vi "svx_DAQ_UpdateMenu.vi"(0 "MenuRef":refnum<k9>, 5 "Display State In":T1={"Channel Info Array"=[], "Timing Mode"=enum."Time", "Timing Control 1"=25600.0, "Timing Control 2"=2560.0, "Timing Control 3"=16, "Timing Indicator 1"=0.1, "Reference Visible?"=FALSE, "Reference Type"=enum."<none>", "Tachometer Channel"="", "Tach Pulses Per Rev"=1, "Tach Direction"=enum."CW", "Tach Slope"=enum."Rising", "Tach Threshold"=0.0, "Trigger Channel"="", "Trigger Level"=20.0, "Pretrigger Samples"=1, "Trigger Slope"=enum."Falling", "Trigger Hysteresis"=0.0, "Logging Visible?"=FALSE, "Enable Logging"=FALSE, "Logfile Path"=path "c:/test.tdms"} caption="State" {"Timing Control 2" format="%#_6f"; "Channel Info Array"."Max" min=0.0 format="± %^#_4g"; "Channel Info Array"."Channel Type" items=["Voltage (V)"=0, "Charge (C)"=9, "-"=99, "SPL (Pa)"=3, "Force (lbf)"=6, "Force (N)"=1, "Acceleration (g) - IEPE"=2, "Acceleration (g) - Charge"=12, "Acceleration (g) - 4 wire DC Voltage"=22, "Velocity (in/s)"=7, "Velocity (mm/s)"=8, "Prox Probe (mil)"=4, "Prox Probe (mm)"=5]}, 11 "error in (no error)":errorcluster) -> (15 "error out":errorcluster)   [LabVIEW 2017, in "SVX NI-DAQmx AI Configuration XControl.xctl"]
uses:
  <vilib>/addons/Sound and Vibration/svt_DAQmx/Configuration XControl/SVX NI-DAQmx AI Configuration XControl.xctl
  <vilib>/addons/Sound and Vibration/svt_DAQmx/Configuration XControl/SubVIs/svx_DAQ_State.ctl
  <vilib>/addons/Sound and Vibration/svt_DAQmx/Configuration XControl/Controls/svx_DAQ_ChannelInfo.ctl
  <vilib>/addons/Sound and Vibration/svt_DAQmx/Configuration XControl/Controls/svx_DAQ_ChannelType.ctl
  <vilib>/addons/Sound and Vibration/svt_DAQmx/Configuration XControl/Controls/svx_DAQ_Coupling.ctl
  <vilib>/addons/Sound and Vibration/svt_DAQmx/Configuration XControl/Controls/svx_DAQ_Excitation.ctl
  <vilib>/addons/Sound and Vibration/svt_DAQmx/Configuration XControl/Controls/svx_DAQ_TimingType.ctl
  <vilib>/addons/Sound and Vibration/svt_DAQmx/Configuration XControl/Controls/svx_DAQ_ReferenceType.ctl
  <vilib>/addons/Sound and Vibration/svt_DAQmx/Configuration XControl/Controls/svx_DAQ_RotationDirection.ctl
  <vilib>/addons/Sound and Vibration/svt_DAQmx/Configuration XControl/Controls/svx_DAQ_Tach_Slope.ctl
  <vilib>/addons/Sound and Vibration/svt_DAQmx/Configuration XControl/Controls/svx_DAQ_Trigger_Slope.ctl
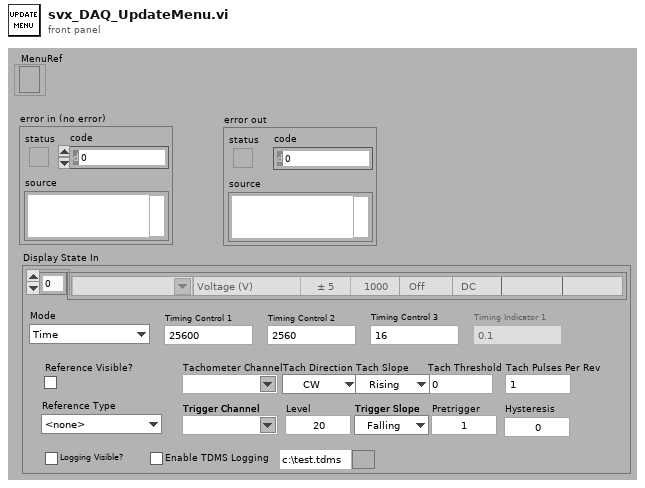
[diagram p1: front panel]
types:
  T1 = typedef "SVX NI-DAQmx AI Configuration XControl.xctl/svx_DAQ_State.ctl" = cluster{"Channel Info Array":T2[], "Timing Mode":T6, "Timing Control 1":dbl, "Timing Control 2":dbl, "Timing Control 3":i32, "Timing Indicator 1":dbl, "Reference Visible?":bool, "Reference Type":T7, "Tachometer Channel":string, "Tach Pulses Per Rev":i32, "Tach Direction":T8, "Tach Slope":T9, "Tach Threshold":dbl, "Trigger Channel":string, "Trigger Level":dbl, "Pretrigger Samples":i32, "Trigger Slope":T10, "Trigger Hysteresis":dbl, "Logging Visible?":bool, "Enable Logging":bool, "Logfile Path":path}
  T2 = typedef "SVX NI-DAQmx AI Configuration XControl.xctl/svx_DAQ_ChannelInfo.ctl" = cluster{"Initialized?":bool, "DAQmx Channel":tag, "Channel Type":T3, "Max":dbl, "Sensitivity":dbl, "Excitation":bool, "Coupling":T4, "Location":string, "Orientation":string, "excitation":T5}
  T3 = typedef "SVX NI-DAQmx AI Configuration XControl.xctl/svx_DAQ_ChannelType.ctl" = u16
  T4 = typedef "SVX NI-DAQmx AI Configuration XControl.xctl/svx_DAQ_Coupling.ctl" = enum16{"AC", "DC"}
  T5 = typedef "svx_DAQ_Excitation.ctl" = enum16{"Off", "Min", "Max"}
  T6 = typedef "SVX NI-DAQmx AI Configuration XControl.xctl/svx_DAQ_TimingType.ctl" = enum16{"Time", "Frequency", "Order"}
  T7 = typedef "SVX NI-DAQmx AI Configuration XControl.xctl/svx_DAQ_ReferenceType.ctl" = enum16{"<none>", "Analog Tachometer", "Analog SW Trigger"}
  T8 = typedef "SVX NI-DAQmx AI Configuration XControl.xctl/svx_DAQ_RotationDirection.ctl" = enum16{"CW", "CCW"}
  T9 = typedef "SVX NI-DAQmx AI Configuration XControl.xctl/svx_DAQ_Tach_Slope.ctl" = enum16{"Rising", "Falling"}
  T10 = typedef "SVX NI-DAQmx AI Configuration XControl.xctl/svx_DAQ_Trigger_Slope.ctl" = enum16{"Falling", "Rising"}
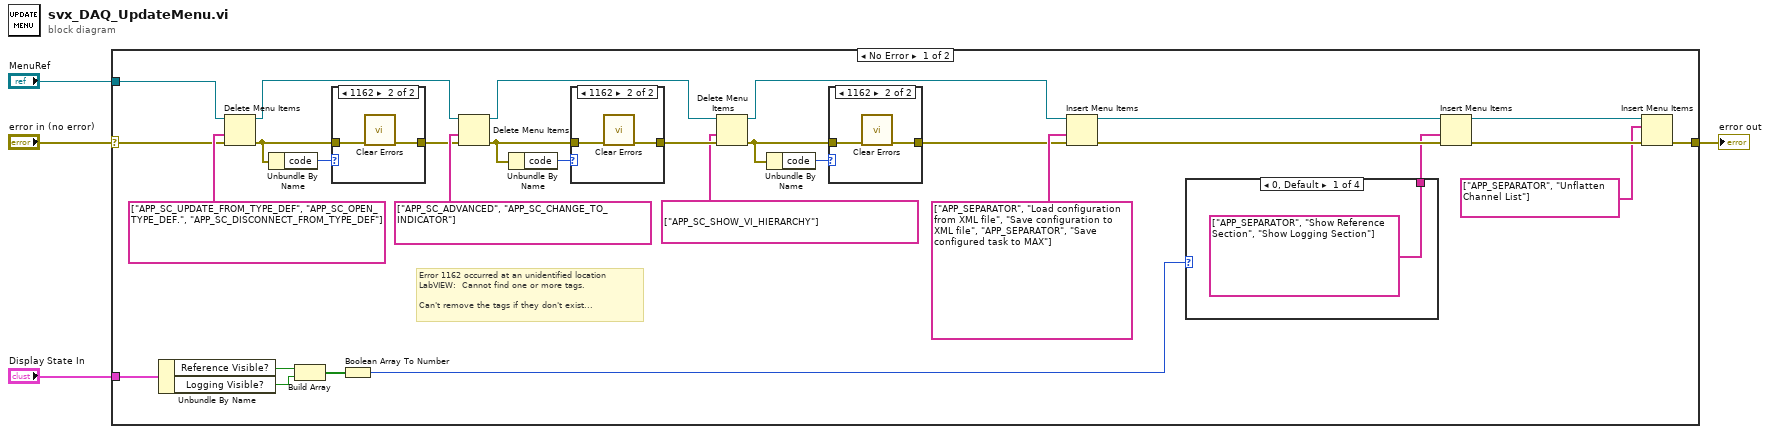
[diagram p0: block diagram]
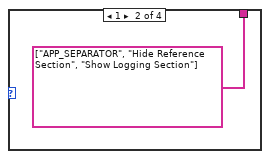
[diagram p2: hidden frame]
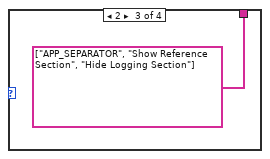
[diagram p3: hidden frame]
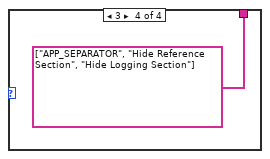
[diagram p4: hidden frame]
diagram:
  n1 = case shown="No Error" "error in (no error)" {
    selector: "error in (no error)" -> [w26 w48]
    tunnel: "MenuRef" -> [w31 _]
    tunnel: [w7 w48] -> w3
    tunnel: "Display State In" -> [w14 _]
    frame No Error {
      # "Error 1162 occurred at an unidentified location\nLabVIEW:  Cannot find one or more tags.\n\nCan't remove the tags if they don't exist..."
      n2 = Unbundle By Name(w14) -> ("Reference Visible?"=w13:bool, "Logging Visible?"=w12:bool)
      n3 = Delete Menu Items(6:w26, 7:string[] ["APP_SC_UPDATE_FROM_TYPE_DEF", "APP_SC_OPEN_TYPE_DEF.", "APP_SC_DISCONNECT_FROM_TYPE_DEF"] ("item tags"), 9:w31) -> (0:w28:errorcluster, 3:w33:refnum<k9>)  [unwired: 1 in]
      n4 = Unbundle By Name(w28) -> ("code"=w29:i32)
      n5 = Build Array(w13, w12) -> (w11:bool[])
      n6 = case shown="1162" w29 {
        tunnel: w28 -> [w45 w47]
        tunnel: [w45 w46] -> w27
        frame 0, Default {
        }
        frame 1162 {
          n7 = call <vilib>:"Clear Errors.vi"("error in (no error)"=w47) -> ("error out"=w46:errorcluster)  [unwired: 5 in, 1 out]
        }
      }
      n8 = Boolean Array To Number(Boolean array=w11) -> (number=w10:u32)
      n9 = Delete Menu Items(6:w27, 7:string[] ["APP_SC_ADVANCED", "APP_SC_CHANGE_TO_INDICATOR"] ("item tags"), 9:w33) -> (0:w25:errorcluster, 3:w20:refnum<k9>)  [unwired: 1 in]
      n10 = Unbundle By Name(w25) -> ("code"=w24:i32)
      n11 = case shown="1162" w24 {
        tunnel: w25 -> [w42 w44]
        tunnel: [w42 w43] -> w21
        frame 0, Default {
        }
        frame 1162 {
          n12 = call <vilib>:"Clear Errors.vi"("error in (no error)"=w44) -> ("error out"=w43:errorcluster)  [unwired: 5 in, 1 out]
        }
      }
      n13 = Delete Menu Items(6:w21, 7:string[] ["APP_SC_SHOW_VI_HIERARCHY"] ("item tags"), 9:w20) -> (0:w22:errorcluster, 3:w16:refnum<k9>)  [unwired: 1 in]
      n14 = Unbundle By Name(w22) -> ("code"=w23:i32)
      n15 = case shown="1162" w23 {
        tunnel: w22 -> [w39 w41]
        tunnel: [w39 w40] -> w18
        frame 0, Default {
        }
        frame 1162 {
          n16 = call <vilib>:"Clear Errors.vi"("error in (no error)"=w41) -> ("error out"=w40:errorcluster)  [unwired: 5 in, 1 out]
        }
      }
      n17 = Insert Menu Items(6:w18, 7:string[] ["APP_SEPARATOR", "Load configuration from XML file", "Save configuration to XML file", "APP_SEPARATOR", "Save configured task to MAX"] ("item tags"), 9:w16) -> (0:w17:errorcluster, 3:w15:refnum<k9>)  [unwired: 3 in, 1 out]
      n18 = case shown="0, Default" w10 {
        tunnel: [string[] ["APP_SEPARATOR", "Show Reference Section", "Show Logging Section"] ("item tags") string[] ["APP_SEPARATOR", "Hide Reference Section", "Show Logging Section"] ("item tags") string[] ["APP_SEPARATOR", "Show Reference Section", "Hide Logging Section"] ("item tags") string[] ["APP_SEPARATOR", "Hide Reference Section", "Hide Logging Section"] ("item tags")] -> w9
        frame 0, Default {
        }
        frame 1 {
        }
        frame 2 {
        }
        frame 3 {
        }
      }
      n19 = Insert Menu Items(6:w17, 7:w9, 9:w15) -> (0:w8:errorcluster, 3:w6:refnum<k9>)  [unwired: 3 in, 1 out]
      n20 = Insert Menu Items(6:w8, 8:string[] ["APP_SEPARATOR", "Unflatten Channel List"] ("item names"), 9:w6) -> (0:w7:errorcluster)  [unwired: 3 in, 2 out]
    }
    frame Error {
    }
  }
  "error out" <- w3
